vi "Do.vi"(8 "error in (no error)":errorcluster, 10 "Actor in":refnum<class "Actor.lvclass">, 11 "Configure Trigger Source [TRG] Msg":refnum<class "Configure Trigger Source [TRG] Msg.lvclass">) -> (0 "error out":errorcluster, 2 "Actor out":refnum<class "Actor.lvclass">)   [LabVIEW 2015, in "CS++DCPwr.lvlib" / "Configure Trigger Source [TRG] Msg.lvclass"]
doc: "This VI delivers the message to the actor by calling the appropriate method(s) on the actor."
uses:
  Configure Trigger Source [TRG] Msg.lvclass
  CS++DCPwr/CS++DCPwr.lvclass
  <vilib>/ActorFramework/Actor/Actor.lvclass
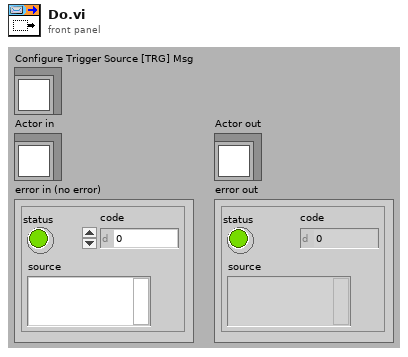
[diagram p1: front panel]
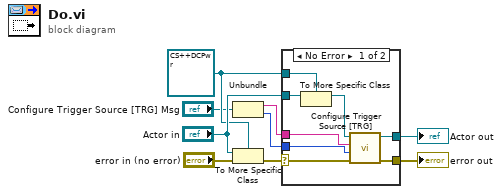
[diagram p0: block diagram]
diagram:
  w4 = refnum<class "CS++DCPwr.lvclass"> refnum ("Actor in")
  n1 = Unbundle ("Main-Unbundle")("Configure Trigger Source [TRG] Msg") -> (w2:string, w1:i32)
  n2 = To More Specific Class(target class=w4, reference="Actor in", error in="error in (no error)") -> (error out=w8:errorcluster)  [unwired: 1 out]
  n3 = case shown="No Error" w8 {
    selector: w8 -> [w15 w19]
    tunnel: [w17 w19] -> w7
    tunnel: [w16 w18] -> w6
    tunnel: "Actor in" -> [w14 w18]
    tunnel: w4 -> [w13 _]
    tunnel: w2 -> [w11 _]
    tunnel: w1 -> [w10 _]
    frame No Error {
      n4 = To More Specific Class(target class=w13, reference=w14) -> (specific class reference=w12:refnum<class "CS++DCPwr.lvclass">)  [unwired: 1 in, 1 out]
      n5 = call "Configure Trigger Source [TRG].vi"("error in (no error)"=w15, "source (Immediate)"=w10, "channel name (\"CHANNEL1\")"=w11, "CS++DCPwr in"=w12) -> ("error out"=w17:errorcluster, "CS++DCPwr out"=w16:refnum<class "CS++DCPwr.lvclass">)  [unwired: 6 in]
    }
    frame Error {
    }
  }
  "error out" <- w7
  "Actor out" <- w6
